vi "Relay output states.vi"() -> ()   [LabVIEW 2013]
panel:
  in  "Byte 2":u8
  in  "Byte 1":u8
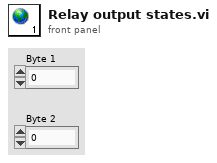
[diagram p1: front panel]
diagram:
